vi "Read Size.vi"(11 "Goal post in":refnum<class "Goal Post.lvclass">) -> (2 "Size":dbl)   [LabVIEW 2021, in "Goal Post.lvclass"]
doc: "MIT Licence\nCopyright (c) 2024 David Grollier"
uses:
  Goal Post.lvclass
  Goal Post.lvclass/Goal Post.ctl
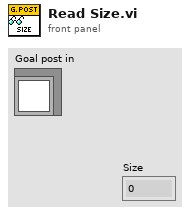
[diagram p1: front panel]
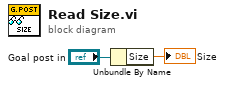
[diagram p0: block diagram]
diagram:
  n1 = Unbundle By Name("Goal post in") -> ("Size"=→"Size":dbl)
